vi "ROI Handler.vi"(0 "IntGraph REF":refnum<vi>, 2 "ROI Action":T1, 7 "X Width (PX)":dbl, 11 "Y Width (PX)":dbl) -> (4 "Graph REF":refnum<vi>, 8 "ROI Indices OUT":i32[][](array[numeric]))   [LabVIEW 2014]
uses:
  ROI Action.ctl
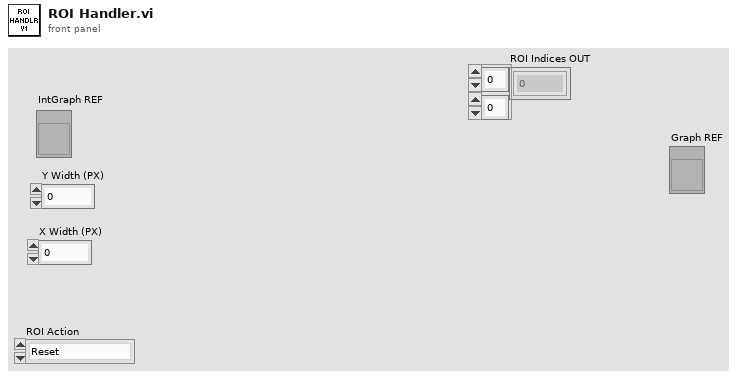
[diagram p1: front panel]
types:
  T1 = typedef "ROI Action.ctl" = enum16{"Reset", "Add New ROI", "Resize ROIs", "Get ROI Indices"}
  T2 = typedef "LVRectTypeDef.ctl" = cluster{"Left":i16, "Top":i16, "Right":i16, "Bottom":i16}
  T3 = typedef "LVPoint32TypeDef.ctl" = cluster{"Horizontal":i32, "Vertical":i32}
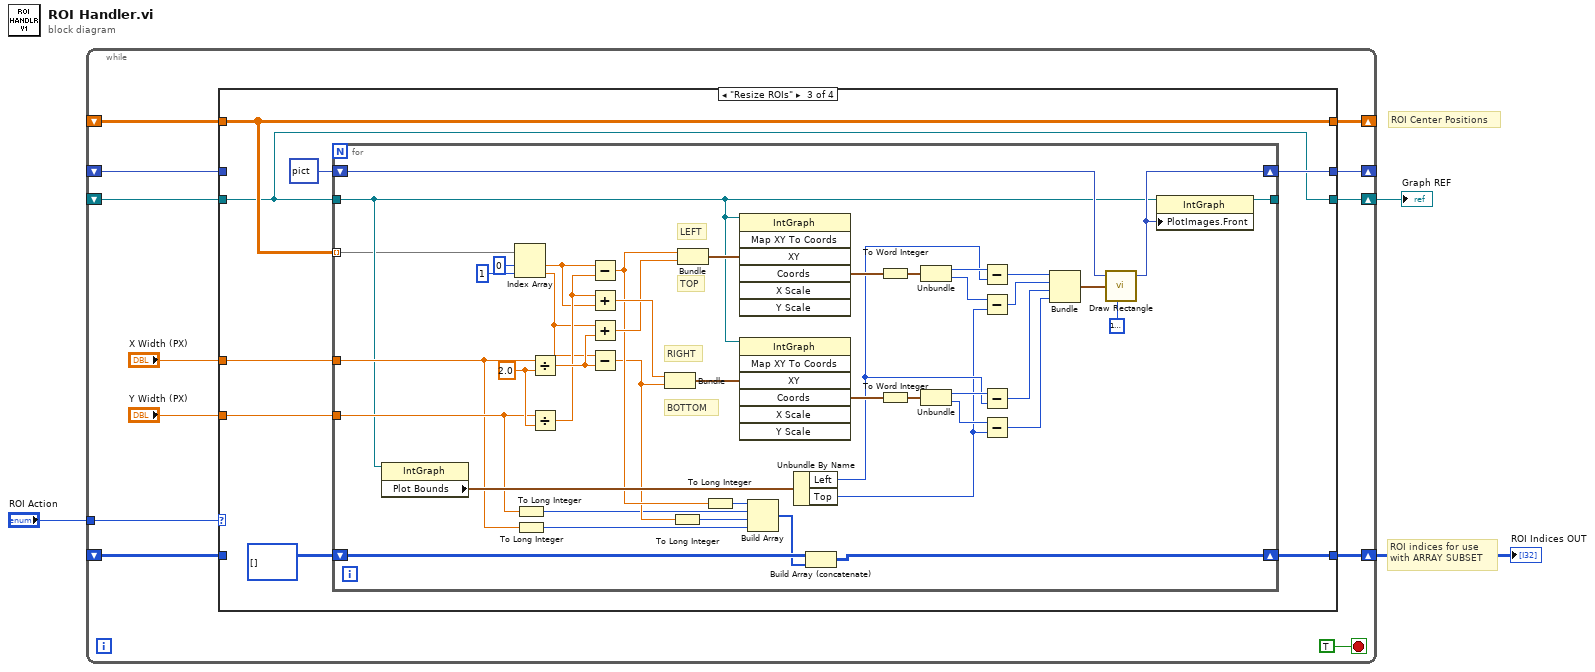
[diagram p0: block diagram]
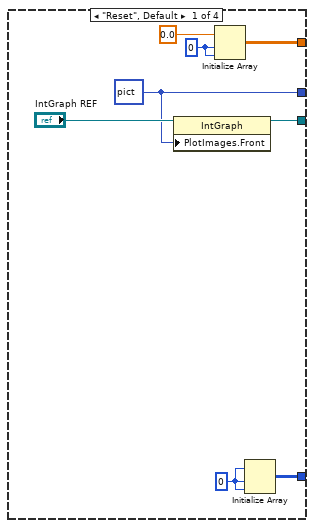
[diagram p2: hidden frame]
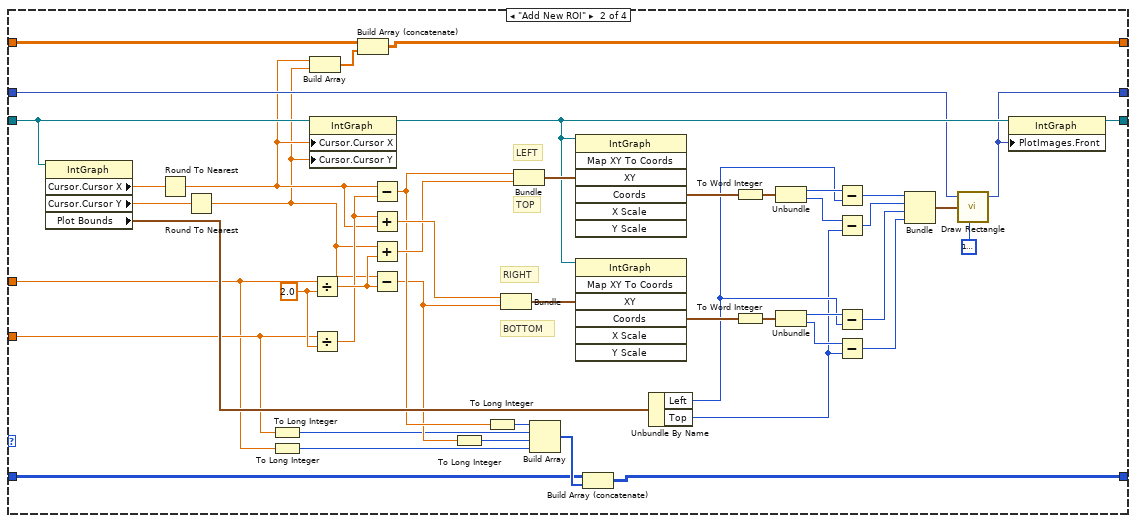
[diagram p3: hidden frame]
diagram:
  # "ROI Center Positions"
  # "ROI indices for use\nwith ARRAY SUBSET"
  n1 = while {
    tunnel: "ROI Action" -> [w15]
    shift-right: [w14] -> _
    shift-left: _ -> [w11]
    shift-right: [w13] -> w1
    shift-left: _ -> [w12]
    shift-right: [w10] -> w2
    shift-left: _ -> [w9]
    shift-right: [w5] -> _
    shift-left: _ -> [w4]
    stop <- TRUE stop-if-true
    n2 = case shown="\"Resize ROIs\"" w15 {
      tunnel: [w19 w29 w76 w125] -> w14
      tunnel: [w20 w37 w71 w124] -> w13
      tunnel: w12 -> [_ w36 w71 w124]
      tunnel: w11 -> [_ w30 _ w125]
      tunnel: [w22 w33 w73 w126] -> w10
      tunnel: w9 -> [_ w34 _ w126]
      tunnel: "Y Width (PX)" -> [_ w32 w78 _]
      tunnel: "X Width (PX)" -> [_ w31 w77 _]
      tunnel: [w16 w24 w75 w123] -> w5
      tunnel: w4 -> [_ w28 w75 w123]
      frame "Reset", Default {
        w18 = 0 ("dimension size")
        w23 = 0 ("dimension size")
        w19 = picture data[5B] ("picture")
        n3 = property class="IntGraph"(reference="IntGraph REF", "PlotImages.Front"=w19) -> (reference out=w20:refnum<vi>)  [unwired: 1 in, 1 out]
        n4 = Initialize Array(0.0 ("element"), w18, w18) -> (w16:dbl[][])
        n5 = Initialize Array(w23, w23, w23) -> (w22:i32[][])
      }
      frame "Add New ROI" {
        w70 = 2.0 ("y")
        # "BOTTOM"
        # "RIGHT"
        # "TOP"
        # "LEFT"
        n6 = property class="IntGraph"(reference=w36) -> ("Cursor.Cursor X"=w69:dbl, "Cursor.Cursor Y"=w68:dbl, "Plot Bounds"=w45:T2)  [unwired: 1 in, 2 out]
        n7 = Round To Nearest(number=w69) -> (nearest integer value=w27:dbl)
        n8 = Round To Nearest(number=w68) -> (nearest integer value=w26:dbl)
        n9 = To Long Integer(number=w32) -> (32bit integer=w38:i32)
        n10 = To Long Integer(number=w31) -> (32bit integer=w40:i32)
        n11 = Build Array(w27, w26) -> (w25:dbl[])
        n12 = property class="IntGraph"(reference=w36, "Cursor.Cursor X"=w27, "Cursor.Cursor Y"=w26) -> (reference out=w42:refnum<vi>)  [unwired: 1 in, 1 out]
        n13 = Divide(x=w31, y=w70) -> (x/y=w49:dbl)
        n14 = Divide(x=w32, y=w70) -> (x/y=w48:dbl)
        n15 = Build Array (concatenate)(w28, w25) -> (w24:dbl[][])
        n16 = Subtract(x=w27, y=w48) -> (x-y=w44:dbl)
        n17 = Add(x=w48, y=w27) -> (x+y=w47:dbl)
        n18 = Add(x=w26, y=w49) -> (x+y=w46:dbl)
        n19 = Subtract(x=w26, y=w49) -> (x-y=w43:dbl)
        n20 = To Long Integer(number=w43) -> (32bit integer=w39:i32)
        n21 = To Long Integer(number=w44) -> (32bit integer=w41:i32)
        n22 = Bundle(w47, w43) -> (w64:cluster{dbl, dbl})  [unwired: 1 in]
        n23 = Bundle(w44, w46) -> (w65:cluster{dbl, dbl})  [unwired: 1 in]
        n24 = Build Array(w41, w38, w39, w40) -> (w35:i32[])
        n25 = invoke class="IntGraph" method="Map XY To Coords"(reference=w42, "XY"=w65) -> ("Coords"=w67:T3)  [unwired: 5 in, 6 out]
        n26 = invoke class="IntGraph" method="Map XY To Coords"(reference=w42, "XY"=w64) -> ("Coords"=w66:T3)  [unwired: 5 in, 6 out]
        n27 = Build Array (concatenate)(w34, w35) -> (w33:i32[][])
        n28 = Unbundle By Name(w45) -> ("Left"=w51:i16, "Top"=w50:i16)
        n29 = To Word Integer(number=w67) -> (16bit integer=w63:cluster{"Horizontal":i16, "Vertical":i16})
        n30 = To Word Integer(number=w66) -> (16bit integer=w62:cluster{"Horizontal":i16, "Vertical":i16})
        n31 = Unbundle(w63) -> ("Horizontal"=w59:i16, "Vertical"=w57:i16)
        n32 = Unbundle(w62) -> ("Horizontal"=w55:i16, "Vertical"=w53:i16)
        n33 = Subtract(x=w59, y=w51) -> (x-y=w58:i16)
        n34 = Subtract(x=w57, y=w50) -> (x-y=w56:i16)
        n35 = Subtract(x=w55, y=w51) -> (x-y=w54:i16)
        n36 = Subtract(x=w53, y=w50) -> (x-y=w52:i16)
        n37 = Bundle(w58, w56, w54, w52) -> (w61:cluster{i16, i16, i16, i16})  [unwired: 1 in]
        n38 = call <vilib>:"Draw Rectangle.vi"("picture"=w30, "rect"=w61, "color(black)"=u32 16777226) -> ("new picture"=w29:picture)  [unwired: 6 in]
        n39 = property class="IntGraph"(reference=w42, "PlotImages.Front"=w29) -> (reference out=w37:refnum<vi>)  [unwired: 1 in, 1 out]
      }
      frame "Resize ROIs" {
        n40 = for {
          tunnel: [w92] -> _
          tunnel: w78 -> [w91]
          tunnel: w77 -> [w90]
          tunnel: w71 -> [w87]
          tunnel: w75 -> [w86] mode=indexing
          shift-right: [w79] -> w73
          shift-left: i32[][] [] -> [w81]
          shift-right: [w88] -> w76
          shift-left: picture data[5B] ("picture") -> [w89]
          w122 = 2.0 ("y")
          # "BOTTOM"
          # "RIGHT"
          # "TOP"
          # "LEFT"
          n41 = property class="IntGraph"(reference=w87) -> ("Plot Bounds"=w99:T2)  [unwired: 1 in, 2 out]
          n42 = Index Array(array=w86, index #1=0 ("index"), index #2=1 ("index")) -> (element #1=w82:dbl, element #2=w83:dbl)
          n43 = To Long Integer(number=w91) -> (32bit integer=w93:i32)
          n44 = To Long Integer(number=w90) -> (32bit integer=w95:i32)
          n45 = Divide(x=w90, y=w122) -> (x/y=w103:dbl)
          n46 = Divide(x=w91, y=w122) -> (x/y=w102:dbl)
          n47 = Subtract(x=w82, y=w102) -> (x-y=w98:dbl)
          n48 = Add(x=w102, y=w82) -> (x+y=w101:dbl)
          n49 = Add(x=w83, y=w103) -> (x+y=w100:dbl)
          n50 = Subtract(x=w83, y=w103) -> (x-y=w97:dbl)
          n51 = Bundle(w101, w97) -> (w118:cluster{dbl, dbl})  [unwired: 1 in]
          n52 = To Long Integer(number=w97) -> (32bit integer=w94:i32)
          n53 = Bundle(w98, w100) -> (w119:cluster{dbl, dbl})  [unwired: 1 in]
          n54 = To Long Integer(number=w98) -> (32bit integer=w96:i32)
          n55 = invoke class="IntGraph" method="Map XY To Coords"(reference=w87, "XY"=w119) -> ("Coords"=w121:T3)  [unwired: 5 in, 6 out]
          n56 = invoke class="IntGraph" method="Map XY To Coords"(reference=w87, "XY"=w118) -> ("Coords"=w120:T3)  [unwired: 5 in, 6 out]
          n57 = Build Array(w96, w93, w94, w95) -> (w80:i32[])
          n58 = Unbundle By Name(w99) -> ("Left"=w105:i16, "Top"=w104:i16)
          n59 = Build Array (concatenate)(w81, w80) -> (w79:i32[][])
          n60 = To Word Integer(number=w121) -> (16bit integer=w117:cluster{"Horizontal":i16, "Vertical":i16})
          n61 = To Word Integer(number=w120) -> (16bit integer=w116:cluster{"Horizontal":i16, "Vertical":i16})
          n62 = Unbundle(w117) -> ("Horizontal"=w113:i16, "Vertical"=w111:i16)
          n63 = Unbundle(w116) -> ("Horizontal"=w109:i16, "Vertical"=w107:i16)
          n64 = Subtract(x=w113, y=w105) -> (x-y=w112:i16)
          n65 = Subtract(x=w111, y=w104) -> (x-y=w110:i16)
          n66 = Subtract(x=w109, y=w105) -> (x-y=w108:i16)
          n67 = Subtract(x=w107, y=w104) -> (x-y=w106:i16)
          n68 = Bundle(w112, w110, w108, w106) -> (w115:cluster{i16, i16, i16, i16})  [unwired: 1 in]
          n69 = call <vilib>:"Draw Rectangle.vi"("picture"=w89, "rect"=w115, "color(black)"=u32 16777226) -> ("new picture"=w88:picture)  [unwired: 6 in]
          n70 = property class="IntGraph"(reference=w87, "PlotImages.Front"=w88) -> (reference out=w92:refnum<vi>)  [unwired: 1 in, 1 out]
        }
      }
      frame "Get ROI Indices" {
      }
    }
  }
  "ROI Indices OUT" <- w2
  "Graph REF" <- w1
